vi "imu_read.vi"(9 "VISA resource name":refnum<visa-resource-name>) -> (2 "read buffer":string)   [LabVIEW 2017]
panel:
  out "VISA resource name 2":refnum<visa-resource-name>
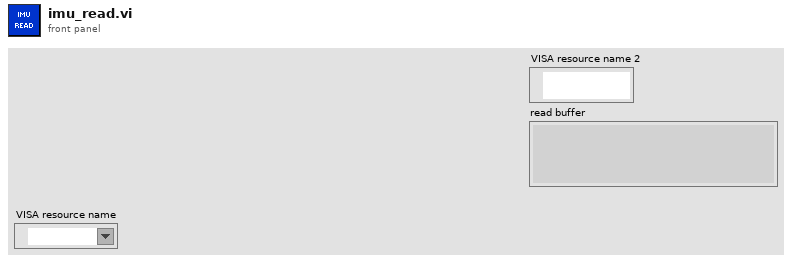
[diagram p1: front panel]
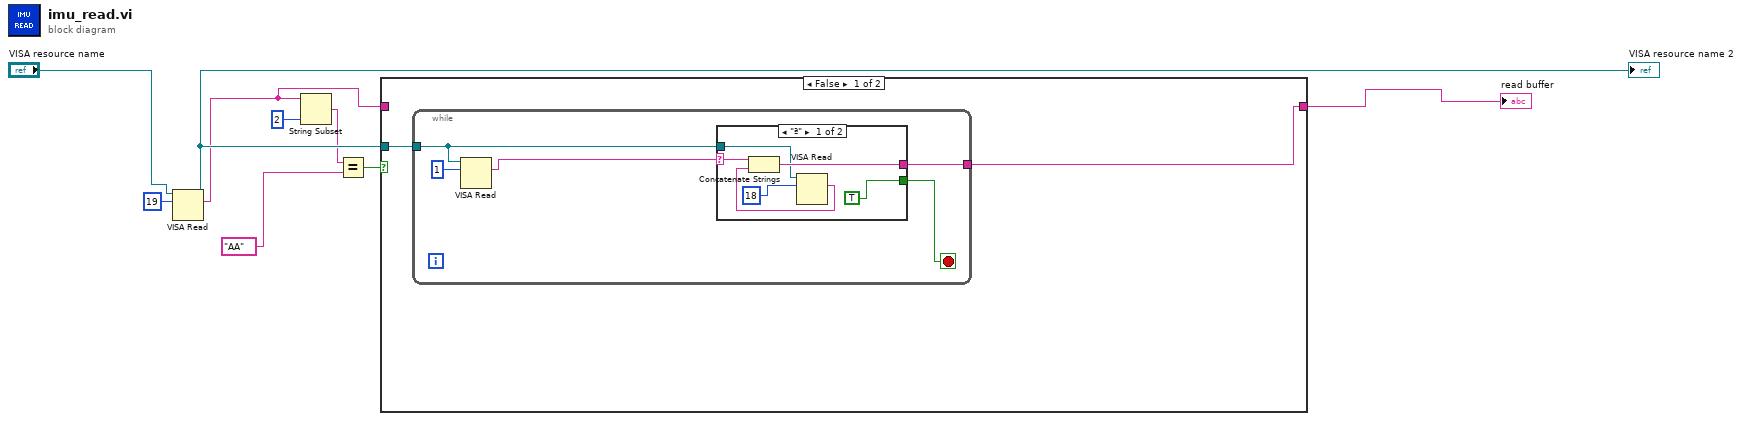
[diagram p0: block diagram]
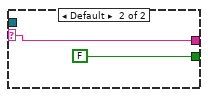
[diagram p2: hidden frame]
diagram:
  n1 = VISA Read(VISA resource name="VISA resource name", byte count=u32 19) -> (VISA resource name out=w7:refnum<visa-resource-name>, read buffer=w1:string)  [unwired: 1 in, 2 out]
  "VISA resource name 2" <- w7
  n2 = String Subset(string=w1, length (rest)=2 ("length (rest)")) -> (substring=w2:string)  [unwired: 1 in]
  n3 = Equal?(x=w2, y="AA") -> (x = y?=w4:bool)
  n4 = case shown="False" w4 {
    tunnel: w1 -> [_ w25]
    tunnel: [w10 w25] -> w8
    tunnel: w7 -> [w11 _]
    frame False {
      n5 = while {
        tunnel: w11 -> [w12]
        tunnel: [w14] -> w10
        stop <- w13 stop-if-true
        n6 = VISA Read(VISA resource name=w12, byte count=u32 1) -> (read buffer=w15:string)  [unwired: 1 in, 3 out]
        n7 = case shown="\"ª\"" w15 {
          selector: w15 -> [w22 w24]
          tunnel: [w20 w24] -> w14
          tunnel: [TRUE FALSE] -> w13
          tunnel: w12 -> [w18 _]
          frame "ª" {
            n8 = VISA Read(VISA resource name=w18, byte count=u32 18) -> (read buffer=w21:string)  [unwired: 1 in, 3 out]
            n9 = Concatenate Strings(w22, w21) -> (w20:string)
          }
          frame Default {
          }
        }
      }
    }
    frame True {
    }
  }
  "read buffer" <- w8
